vi "iWorx - Set Up Utility.vi"() -> ()   [LabVIEW 2012]
uses:
  <vilib>/Utility/file.llb/Write To Spreadsheet File (string).vi
panel:
  out "Files in Sheet":i32
  out "Files on disc":i32
  in  "Directory":path=path "C:/Users/husmith/Documents/Hunter Drive/minisystemtracking.1/iWorx/Code"
  in  "CSV File":path=path "C:/Users/husmith/Documents/Hunter Drive/minisystemtracking.1/iWorx/Documentation/Set Up Instruction Text2.csv"
  out "Array":cluster{"Title":string, "Instructions":string}[](array[cluster])
  in  "Mode":bool
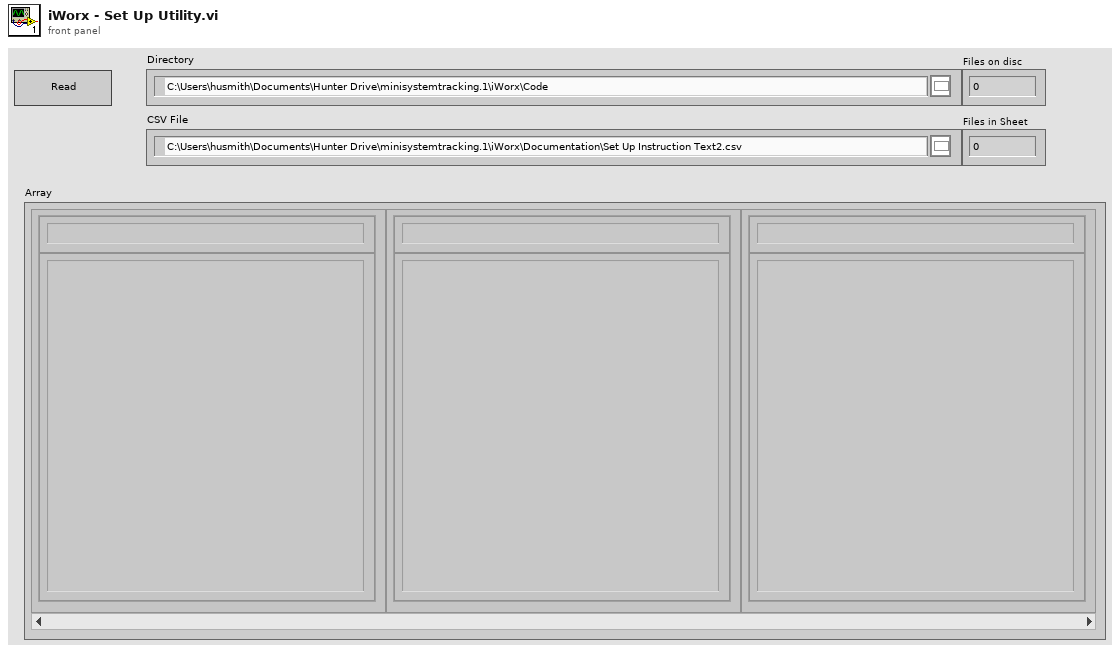
[diagram p1: front panel]
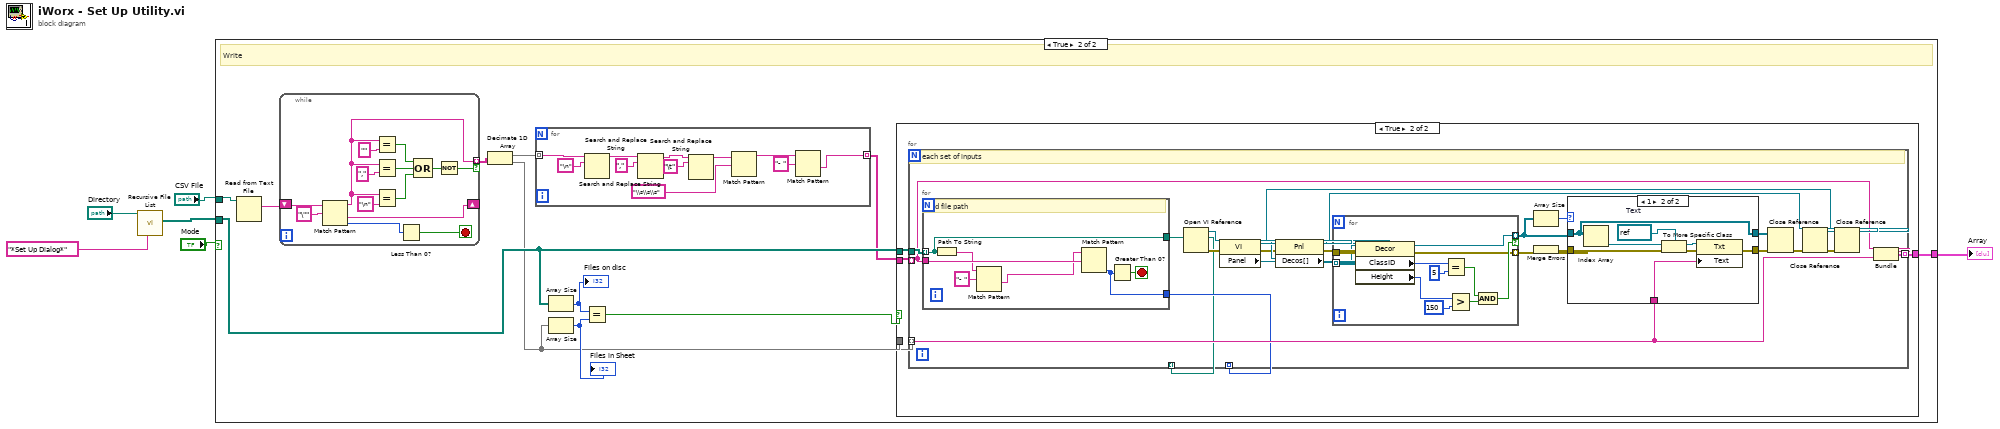
[diagram p0: block diagram]
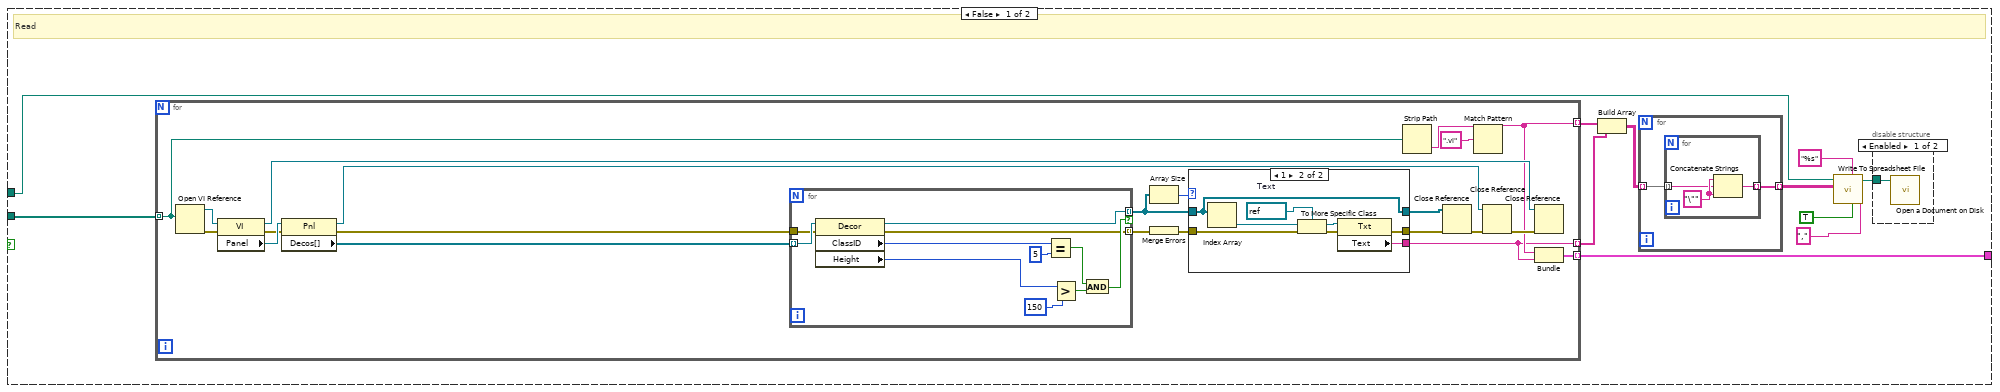
[diagram p2: hidden frame]
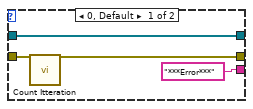
[diagram p4: hidden frame]
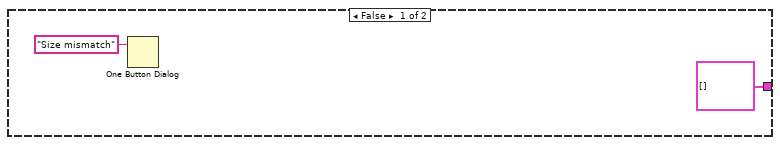
[diagram p5: hidden frame]
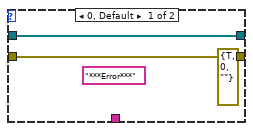
[diagram p6: hidden frame]
diagram:
  n1 = call <vilib>:"Recursive File List.vi"("pattern"="*Set Up Dialog*" ("regular expression"), "Folder Path"="Directory") -> ("All Files in Dir"=w4:path[])  [unwired: 5 in, 4 out]
  n2 = case shown="True" "Mode" {
    tunnel: w4 -> [w9 w74]
    tunnel: "CSV File" -> [w8 w78]
    tunnel: [w7 w76] -> w1
    frame False {
      # "Read"
      n3 = for {
        tunnel: [w25] -> w16 mode=indexing
        tunnel: w9 -> [w29] mode=indexing
        tunnel: [w26] -> w17 mode=indexing
        tunnel: [w24] -> w7 mode=indexing
        n4 = Open VI Reference(vi path=w29) -> (vi reference=w45:refnum<vi>, error out=w44:errorcluster)  [unwired: 5 in]
        n5 = property class="VI"(reference=w45, error in=w44) -> (reference out=w30:refnum<vi>, error out=w39:errorcluster, "Panel"=w43:refnum<vi>)
        n6 = property class="Pnl"(reference=w43, error in=w39) -> (reference out=w32:refnum<vi>, error out=w35:errorcluster, "Decos[]"=w42:refnum<vi>[])
        n7 = for {
          tunnel: w42 -> [w67] mode=indexing
          tunnel: [w66] -> w41 mode=indexing if=w62
          tunnel: [w58] -> w36 mode=indexing
          tunnel: w35 -> [w57]
          n8 = property class="Decor"(reference=w67, error in=w57) -> (reference out=w66:refnum<vi>, error out=w58:errorcluster, "ClassID"=w65:u32, "Height"=w61:u32)
          n9 = Equal?(x=w65, y=u32 5) -> (x = y?=w63:bool)
          n10 = Greater?(x=w61, y=u32 150) -> (0:w59:bool)
          n11 = And(x=w63, y=w59) -> (x .and. y?=w62:bool)
        }
        n12 = Array Size(array=w41) -> (size(s)=w40:i32)
        n13 = Merge Errors(w36) -> (w34:errorcluster)
        n14 = case shown="1" w40 {
          tunnel: w41 -> [w46 w50]
          tunnel: ["***Error***" ("Text") w49] -> w25
          tunnel: [w46 w50] -> w38
          tunnel: [w47 w52] -> w37
          tunnel: w34 -> [w47 w51]
          frame 0, Default {
            n15 = call "Count Itteration.vi"() -> ()  [unwired: 7 in, 2 out]
          }
          frame 1 {
            w55 = refnum<vi> refnum  # Text
            n16 = Index Array(array=w50) -> (element=w56:refnum<vi>)  [unwired: 1 in]
            n17 = To More Specific Class(target class=w55, reference=w56, error in=w51) -> (specific class reference=w54:refnum<vi>, error out=w53:errorcluster)
            n18 = property class="Txt"(reference=w54, error in=w53) -> (error out=w52:errorcluster, "Text"=w49:string)  [unwired: 1 out]
          }
        }
        n19 = Strip Path(path=w29) -> (name=w28:string)  [unwired: 1 out]
        n20 = Close Reference(reference=w38, error in (no error)=w37) -> (error out=w33:errorcluster)
        n21 = Match Pattern(string=w28, regular expression=".vi" ("search string")) -> (before substring=w26:string)  [unwired: 1 in, 3 out]
        n22 = Close Reference(reference=w32, error in (no error)=w33) -> (error out=w31:errorcluster)
        n23 = Close Reference(reference=w30, error in (no error)=w31) -> ()  [unwired: 1 out]
        n24 = Bundle("name"=w26, "Text"=w25) -> (w24:cluster{"name":string, "Text":string})  [unwired: 1 in]
      }
      n25 = Build Array(w17, w16) -> (w15:string[][])
      n26 = for {
        tunnel: w15 -> [w19] mode=indexing
        tunnel: [w18] -> w10 mode=indexing
        n27 = for {
          tunnel: w19 -> [w21] mode=indexing
          tunnel: [w20] -> w18 mode=indexing
          w22 = "\"" ("string")
          n28 = Concatenate Strings(w22, w21, w22) -> (w20:string)
        }
      }
      n29 = call-poly <vilib>:"Write To Spreadsheet File.vi"("delimiter (\\t)"="," ("delimiter (\\t)"), "transpose? (no:F)"=TRUE, "format (%s)"="%s", "2D data"=w10, "file path (dialog if empty)"=w8) -> ("new file path (Not A Path if cancelled)"=w14:path)  [unwired: 3 in]
      n30 = disable-structure shown="Enabled" {
        disable-tunnel: w14 -> [w23 _]
        frame Enabled {
          n31 = call <vilib>:"Open a Document on Disk.vi"("document path"=w23) -> ()  [unwired: 6 in, 1 out]
        }
        frame Disabled {
        }
      }
    }
    frame True {
      # "Write"
      n32 = Read from Text File(file (use dialog)=w78) -> (text=w77:string)  [unwired: 3 in, 3 out]
      n33 = while {
        shift-right: [w157] -> _
        shift-left: w77 -> [w159]
        tunnel: [w146] -> w69 mode=indexing if=w154
        stop <- w147 stop-if-true
        n34 = Match Pattern(string=w159, regular expression="\"") -> (before substring=w146:string, after substring=w157:string, offset past match=w148:i32)  [unwired: 1 in, 1 out]
        n35 = Equal?(x=w146, y="") -> (x = y?=w152:bool)
        n36 = Equal?(x=w146, y=",") -> (x = y?=w150:bool)
        n37 = Equal?(x=w146, y="\n") -> (x = y?=w149:bool)
        n38 = Less Than 0?(x=w148) -> (x < 0?=w147:bool)
        n39 = Compound Arithmetic op=OR(w152, w150, w149) -> (w151:bool)
        n40 = Not(x=w151) -> (.not. x?=w154:bool)
      }
      n41 = Decimate 1D Array(w69) -> (w75:string[], w70:string[])
      n42 = for {
        tunnel: w75 -> [w145] mode=indexing
        tunnel: [w139] -> w68 mode=indexing
        n43 = Search and Replace String(input string=w145, search string="\n") -> (result string=w143:string)  [unwired: 6 in, 3 out]
        n44 = Search and Replace String(input string=w143, search string=",") -> (result string=w135:string)  [unwired: 6 in, 3 out]
        n45 = Search and Replace String(input string=w135, search string="\t") -> (result string=w136:string)  [unwired: 6 in, 3 out]
        n46 = Match Pattern(string=w136, regular expression="\\s\\s\\s") -> (before substring=w140:string)  [unwired: 1 in, 3 out]
        n47 = Match Pattern(string=w140, regular expression="- ") -> (after substring=w139:string)  [unwired: 1 in, 3 out]
      }
      n48 = Array Size(array=w74) -> (size(s)=w73:i32)
      "Files on disc" <- w73
      n49 = Array Size(array=w70) -> (size(s)=w71:i32)
      "Files in Sheet" <- w71
      n50 = Equal?(x=w73, y=w71) -> (x = y?=w72:bool)
      n51 = case shown="True" w72 {
        tunnel: [cluster{"result string":string, string}[] [] w84] -> w76
        tunnel: w68 -> [_ w83]
        tunnel: w70 -> [_ w82]
        tunnel: w74 -> [_ w81]
        frame False {
          n52 = One Button Dialog(message="Size mismatch") -> ()  [unwired: 1 in, 1 out]
        }
        frame True {
          n53 = for {
            tunnel: w81 -> [w106]
            tunnel: [w105] -> w84 mode=indexing
            tunnel: w82 -> [w89] mode=indexing
            tunnel: w83 -> [w88] mode=indexing
            tunnel: [w87] -> _ mode=indexing
            tunnel: [w86] -> _ mode=indexing
            # "for each set of inputs"
            n54 = for {
              tunnel: w106 -> [w133] mode=indexing
              tunnel: [w133] -> w86
              tunnel: w88 -> [w131]
              tunnel: [w132] -> w87
              stop <- w134 stop-if-true
              # "Find file path"
              n55 = Path To String(path=w133) -> (string=w129:string)
              n56 = Match Pattern(string=w129, regular expression="- ") -> (after substring=w128:string)  [unwired: 1 in, 3 out]
              n57 = Match Pattern(string=w128, regular expression=w131) -> (offset past match=w132:i32)  [unwired: 1 in, 3 out]
              n58 = Greater Than 0?(x=w132) -> (x > 0?=w134:bool)
            }
            n59 = Open VI Reference(vi path=w86) -> (vi reference=w104:refnum<vi>, error out=w103:errorcluster)  [unwired: 5 in]
            n60 = property class="VI"(reference=w104, error in=w103) -> (reference out=w90:refnum<vi>, error out=w99:errorcluster, "Panel"=w102:refnum<vi>)
            n61 = property class="Pnl"(reference=w102, error in=w99) -> (reference out=w92:refnum<vi>, error out=w95:errorcluster, "Decos[]"=w101:refnum<vi>[])
            n62 = for {
              tunnel: w101 -> [w127] mode=indexing
              tunnel: [w126] -> w100 mode=indexing if=w122
              tunnel: [w118] -> w96 mode=indexing
              tunnel: w95 -> [w117]
              n63 = property class="Decor"(reference=w127, error in=w117) -> (reference out=w126:refnum<vi>, error out=w118:errorcluster, "ClassID"=w125:u32, "Height"=w121:u32)
              n64 = Equal?(x=w125, y=u32 5) -> (x = y?=w123:bool)
              n65 = Greater?(x=w121, y=u32 150) -> (0:w119:bool)
              n66 = And(x=w123, y=w119) -> (x .and. y?=w122:bool)
            }
            n67 = Array Size(array=w100) -> (size(s)=w85:i32)
            n68 = Merge Errors(w96) -> (w94:errorcluster)
            n69 = case shown="1" w85 {
              tunnel: w100 -> [w107 w112]
              tunnel: [w107 w112] -> w98
              tunnel: [w108 w109] -> w97
              tunnel: w94 -> [w108 w113]
              tunnel: w89 -> [_ w110]
              frame 0, Default {
                (unwired) errorcluster {"status"=TRUE, "code"=0, "source"=""} ("error out")
                (unwired) "***Error***" ("Text")
              }
              frame 1 {
                w115 = refnum<vi> refnum  # Text
                n70 = Index Array(array=w112) -> (element=w116:refnum<vi>)  [unwired: 1 in]
                n71 = To More Specific Class(target class=w115, reference=w116, error in=w113) -> (specific class reference=w111:refnum<vi>, error out=w114:errorcluster)
                n72 = property class="Txt"(reference=w111, error in=w114, "Text"=w110) -> (error out=w109:errorcluster)  [unwired: 1 out]
              }
            }
            n73 = Close Reference(reference=w98, error in (no error)=w97) -> (error out=w93:errorcluster)
            n74 = Close Reference(reference=w92, error in (no error)=w93) -> (error out=w91:errorcluster)
            n75 = Close Reference(reference=w90, error in (no error)=w91) -> ()  [unwired: 1 out]
            n76 = Bundle("result string"=w88, w89) -> (w105:cluster{"result string":string, string})  [unwired: 1 in]
          }
        }
      }
    }
  }
  "Array" <- w1
